vi "Modified Write Characters To File.vi"(0 "convert eol? (no:F)":bool, 6 "append to file? (new file:F)":bool, 7 "pattern":string, 9 "character string":string, 10 "start path  (Not A Path)":path=path "", 11 "file path (dialog if empty)":path) -> (3 "new file path (Not A Path if cancelled)":path)   [LabVIEW 2015]
doc: "Writes a character string to a new byte stream file or appends the string to an existing file. The VI opens or creates the file beforehand and closes it afterwards.\n\nfile path is the path name of the file. If file path is empty (default value) or is Not A Path, the VI displays a File dialog box from which you can select a file. Error 43 occurs if the user cancels the dialog. \n\ncharacter string is the data the VI writes to the file.\n\nappend to file? Set to TRUE if you want to append the data to a existing file; you can also set it TRUE to write to a new file. Set to FALSE (default value) if you want to write the data to a new file or to replace an existing file.\n\nnew file path is the path of the file to which the VI wrote data. You can use this output to determine the path of a file that you open using dialog. new file path returns Not A Path if the user selects Cancel from the dialog box."
panel:
  in  "prompt":string="Choose file to write."
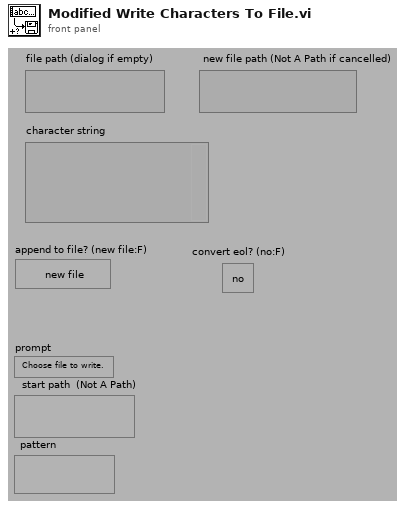
[diagram p1: front panel]
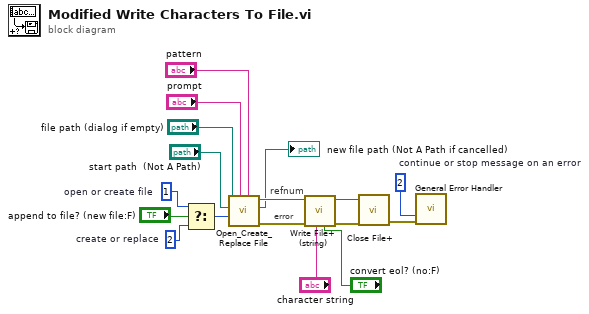
[diagram p0: block diagram]
diagram:
  w7 = i16 2  # create or replace
  w15 = 2  # continue or stop message on an error
  w10 = i16 1  # open or create file
  # "error"
  # "refnum"
  n1 = Select(t=w10, s="append to file? (new file:F)", f=w7) -> (s? t:f=w12:i16)
  n2 = call <vilib>:"Open_Create_Replace File.vi"("pattern"="pattern", "prompt"="prompt", "function (open:0)"=w12, "start path  (Not A Path)"="start path  (Not A Path)", "file path"="file path (dialog if empty)") -> ("error out"=w16:errorcluster, "new file path"=→"new file path (Not A Path if cancelled)":path, "refnum"=w6:refnum<file>)  [unwired: 3 in, 1 out]
  n3 = call <vilib>:"Write File+ (string).vi"("convert eol? (no:F)"="convert eol? (no:F)", "string"="character string", "error in (no error)"=w16, "refnum"=w6) -> ("error out"=w14:errorcluster, "dup refnum"=w13:refnum<file>)  [unwired: 3 in, 1 out]
  n4 = call <vilib>:"Close File+.vi"("error in (no error)"=w14, "refnum"=w13) -> ("error out"=w11:errorcluster)  [unwired: 3 in, 2 out]
  n5 = call <vilib>:"General Error Handler.vi"("type of dialog (OK msg:1)"=w15, "error in (no error)"=w11) -> ()  [unwired: 9 in, 5 out]
